vi "State Machine Kernel.vi"(4 "Init?":bool, 5 "Inputs":T4 {"Kobuki Sensors"."Charger Source" items=["DISCHARGING"=0, "DOCKING_CHARGED"=2, "DOCKING_CHARGING"=6, "ADAPTER_CHARGED"=18, "ADAPTER_CHARGING"=22]; "accelerometer"."z axis (g)" format="%.3f"; "accelerometer"."y axis (g)" format="%.3f"; "accelerometer"."x axis (g)" format="%.3f"}, 7 "StateData In":T1) -> (0 "Terminated?":bool, 2 "Outputs":T3, 3 "StateData Out":T1)   [LabVIEW 2017]
uses:
  controls/Inputs.ctl
  shared/Accelerometer.ctl
  Kobuki/KobukiSensors.ctl
  Kobuki/Kobuki Bumps and WheelDrops.ctl
  Kobuki/Kobuki Buttons.ctl
  controls/Outputs.ctl
  controls/StateData.ctl
  controls/StatesEnum.ctl
panel:
  # "Electrical: charging, battery, OI mode"
  # "Sensors: bump, cliff, button, wheel drop"
  # "Motors:"
  # "Inertia"
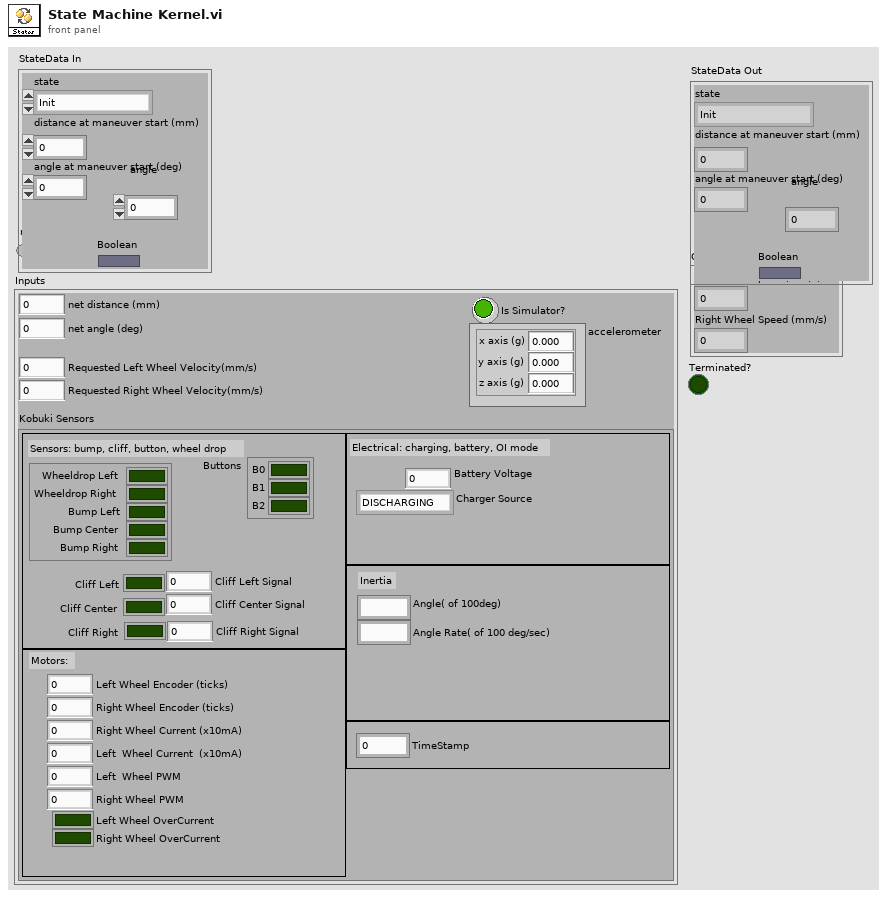
[diagram p1: front panel]
types:
  T1 = typedef "StateData.ctl" = cluster{"distance at maneuver start (mm)":i32, "angle at maneuver start (deg)":i32, "state":T2, "Boolean":bool, "angle":i32}
  T2 = typedef "StatesEnum.ctl" = enum16{"Init", "Center Cliff\n", "Pause", "Drive", "U.Turn", "L.Cliff", "R.Cliff", "Shut", "L.Bump", "R.Bump"}
  T3 = typedef "Outputs.ctl" = cluster{"Left Wheel Speed (mm/s)":i16, "Right Wheel Speed (mm/s)":i16}
  T4 = typedef "Inputs.ctl" = cluster{"net distance (mm)":i32, "net angle (deg)":i32, "accelerometer":T5, "Is Simulator?":bool, "Kobuki Sensors":T6, "Requested Left Wheel Velocity(mm/s)":i32, "Requested Right Wheel Velocity(mm/s)":i32}
  T5 = typedef "Accelerometer.ctl" = cluster{"x axis (g)":dbl, "y axis (g)":dbl, "z axis (g)":dbl}
  T6 = typedef "KobukiSensors.ctl" = cluster{"Bumps + Wheel Drops":T7, "Cliff Left":bool, "Cliff Center":bool, "Cliff Right":bool, "Cliff Left Signal":u16, "Cliff Center Signal":u16, "Cliff Right Signal":u16, "Buttons":T8, "Left Wheel Encoder (ticks)":u16, "Right Wheel Encoder (ticks) ":u16, "Left  Wheel PWM":i8, "Right Wheel PWM":i8, "Left Wheel OverCurrent":bool, "Right Wheel OverCurrent ":bool, "Right Wheel Current (x10mA)":i16, "Left  Wheel Current  (x10mA)":i16, "TimeStamp":u16, "Battery Voltage":dbl, "Angle( of 100deg)":i16, "Angle Rate( of 100 deg/sec)":i16, "Charger Source ":i8}
  T7 = typedef "Kobuki Bumps and WheelDrops.ctl" = cluster{"Wheeldrop Left":bool, "Wheeldrop Right":bool, "Bump Left":bool, "Bump Center":bool, "Bump Right":bool}
  T8 = typedef "Kobuki Buttons.ctl" = cluster{"B0":bool, "B1":bool, "B2":bool}
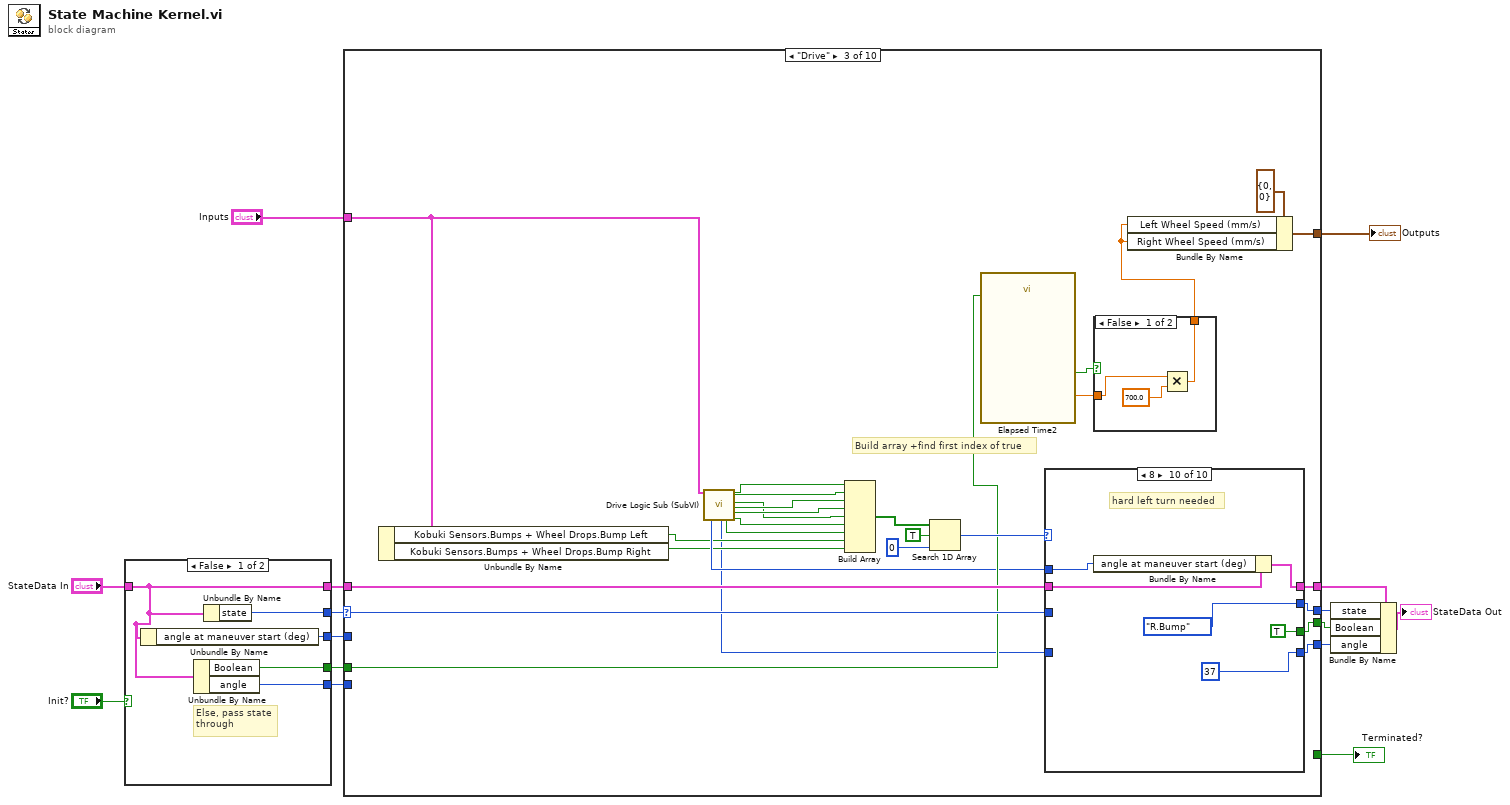
[diagram p0: block diagram]
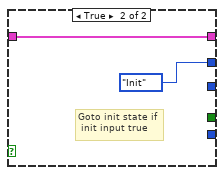
[diagram p2: hidden frame]
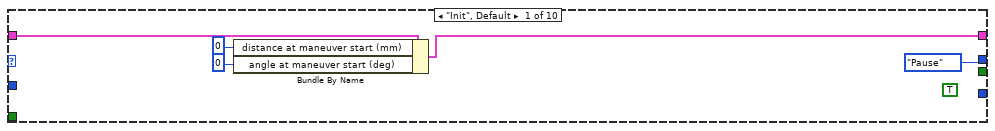
[diagram p3: hidden frame]
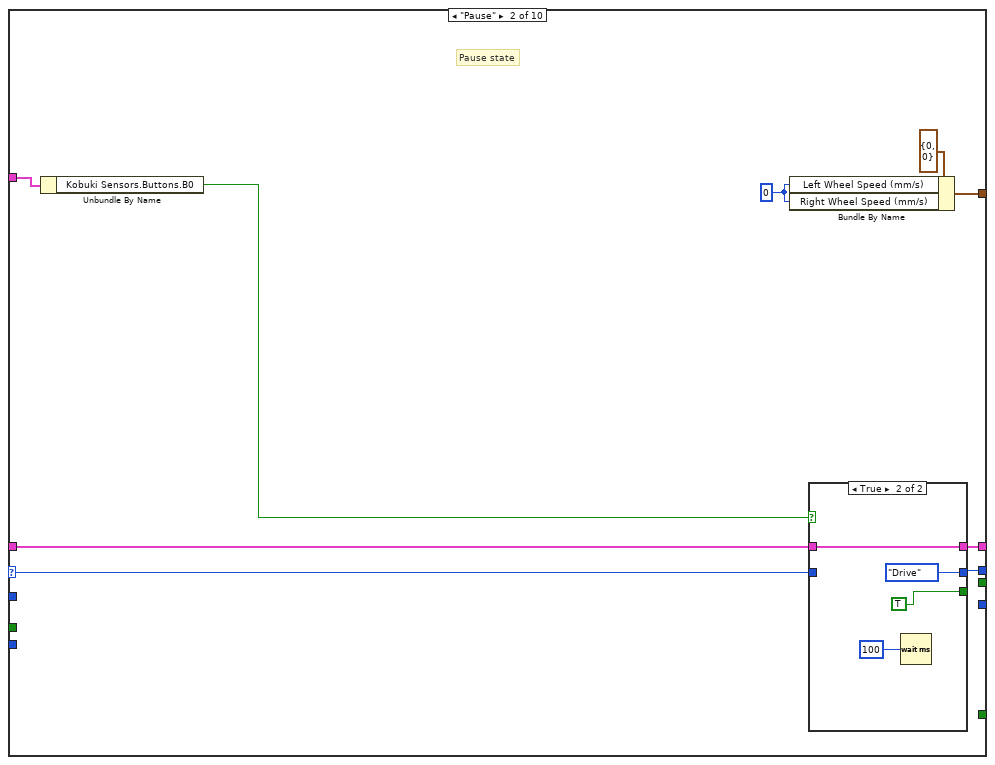
[diagram p4: hidden frame]
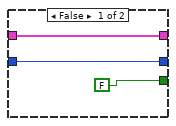
[diagram p5: hidden frame]
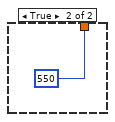
[diagram p6: hidden frame]
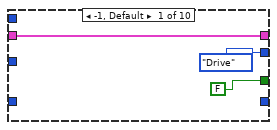
[diagram p7: hidden frame]
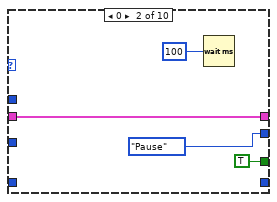
[diagram p8: hidden frame]
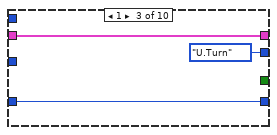
[diagram p9: hidden frame]
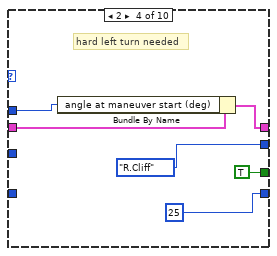
[diagram p10: hidden frame]
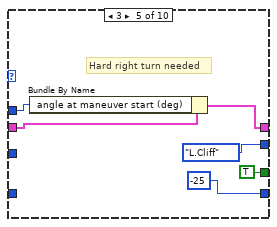
[diagram p11: hidden frame]
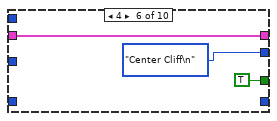
[diagram p12: hidden frame]
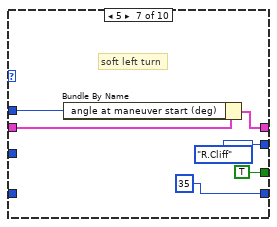
[diagram p13: hidden frame]
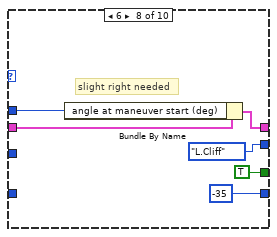
[diagram p14: hidden frame]
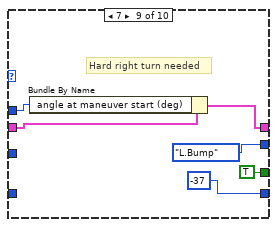
[diagram p15: hidden frame]
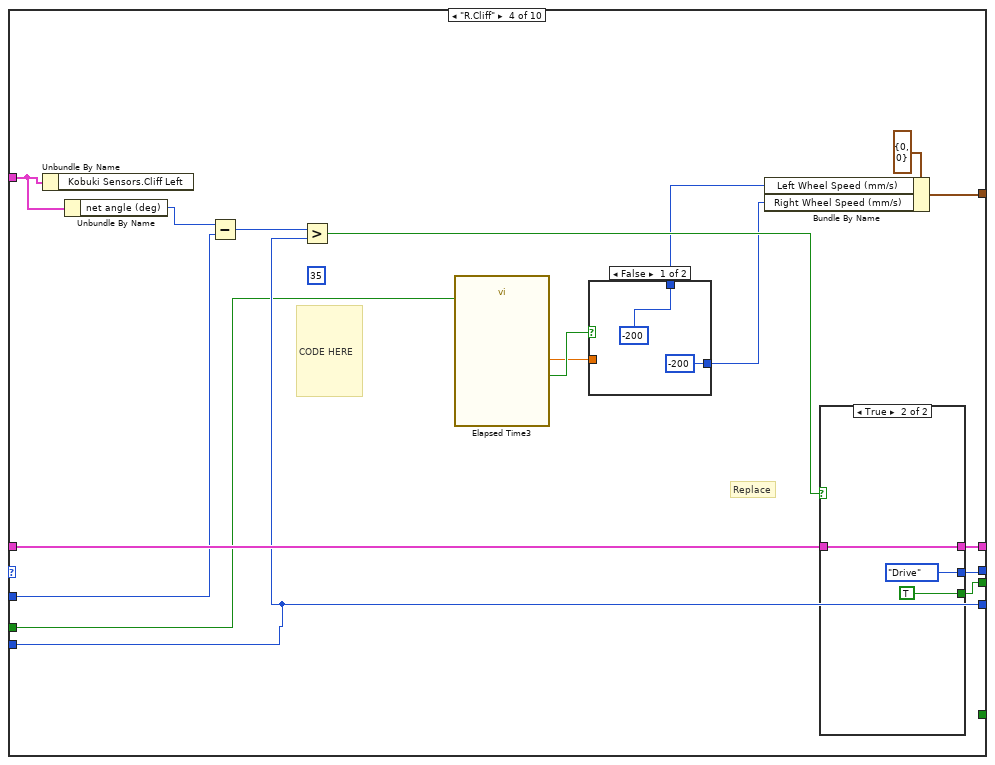
[diagram p16: hidden frame]
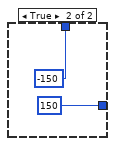
[diagram p17: hidden frame]
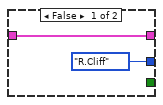
[diagram p18: hidden frame]
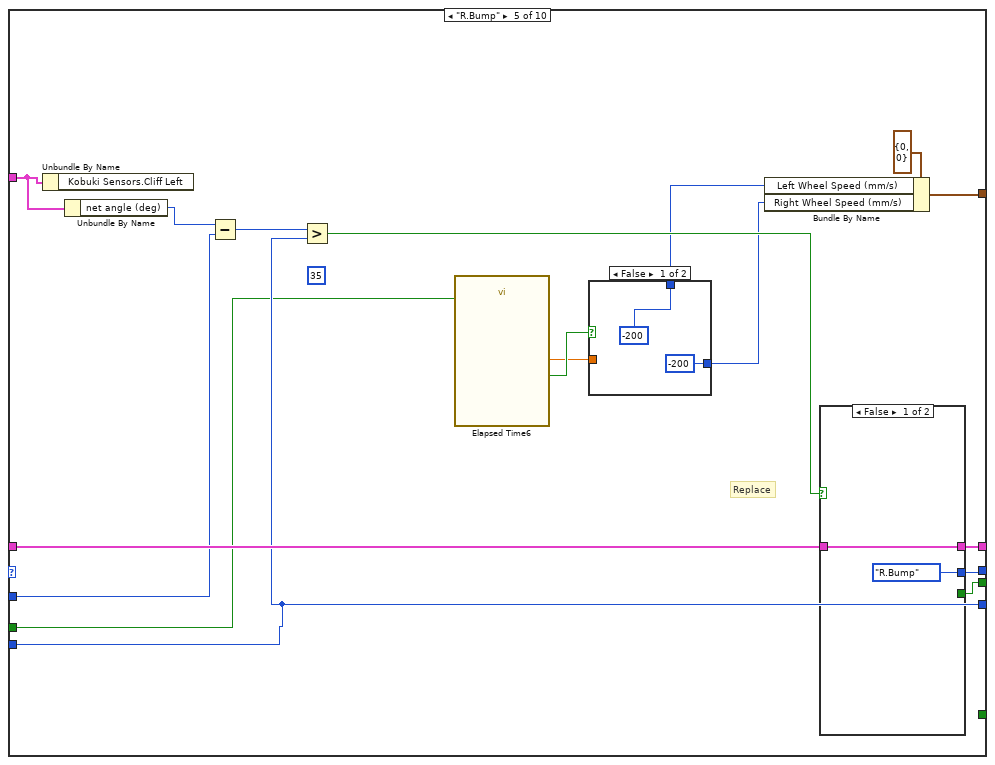
[diagram p19: hidden frame]
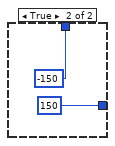
[diagram p20: hidden frame]
diagram:
  n1 = case shown="False" "Init?" {
    tunnel: [w20 StatesEnum."Init" ("StateIn")] -> w13
    tunnel: "StateData In" -> [w18 w21]
    tunnel: [w18 w21] -> w9
    tunnel: [w19 _] -> w6
    tunnel: [w17 _] -> w5
    tunnel: [w16 _] -> w2
    frame False {
      # "Else, pass state \nthrough"
      n2 = Unbundle By Name(w18) -> ("angle at maneuver start (deg)"=w19:i32)
      n3 = Unbundle By Name(w18) -> ("Boolean"=w17:bool, "angle"=w16:i32)
      n4 = Unbundle By Name(w18) -> ("state"=w20:T2)
    }
    frame True {
      # "Goto init state if\n init input true"
    }
  }
  n5 = case shown="\"Drive\"" w13 {
    selector: w13 -> [_ w32 w71 _ _ _ _ _ _ w287]
    tunnel: "Inputs" -> [_ w33 w47 w135 w161 w189 w218 w246 w272 _]
    tunnel: [_ w36 w69 w140 w166 w192 w221 w244 w275 w290] -> w11
    tunnel: [_ _ _ _ _ _ _ _ _ TRUE] -> w12
    tunnel: w9 -> [w27 w30 w64 w138 w164 w190 w219 w242 w273 w288]
    tunnel: [w26 w29 w63 w139 w165 w191 w220 w241 w274 w288] -> w8
    tunnel: w6 -> [_ _ _ w134 w160 w187 w216 _ w270 _]
    tunnel: w5 -> [_ _ w62 w127 w153 w179 w208 w235 _ _]
    tunnel: [_ _ w57 w131 w157 w183 w212 w240 w267 _] -> w4
    tunnel: [StatesEnum."Pause" ("StateIn") w28 w58 w132 w158 w184 w213 w239 w268 w287] -> w3
    tunnel: w2 -> [_ _ _ w130 w156 w182 w211 _ w260 _]
    tunnel: [_ _ w56 w130 w156 w182 w211 _ w260 _] -> w1
    frame "Init", Default {
      (unwired) TRUE
      n6 = Bundle By Name(cluster=w27, "distance at maneuver start (mm)"=0, "angle at maneuver start (deg)"=0) -> (w26:T1)
    }
    frame "Pause" {
      w35 = i16 0 ("Left Wheel Speed (mm/s)")
      # "Pause state"
      n7 = Unbundle By Name(w33) -> ("Kobuki Sensors.Buttons.B0"=w34:bool)
      n8 = Bundle By Name(cluster=T3 {"Left Wheel Speed (mm/s)"=0, "Right Wheel Speed (mm/s)"=0} ("Outputs"), "Left Wheel Speed (mm/s)"=w35, "Right Wheel Speed (mm/s)"=w35) -> (w36:T3)
      n9 = case shown="True" w34 {
        tunnel: w32 -> [w39 _]
        tunnel: [w39 StatesEnum."Drive" ("StateIn")] -> w28
        tunnel: w30 -> [w38 w41]
        tunnel: [w38 w41] -> w29
        tunnel: [FALSE TRUE] -> _
        frame False {
        }
        frame True {
          n10 = Wait (ms)(milliseconds to wait=u32 100) -> ()  [unwired: 1 out]
        }
      }
    }
    frame "Drive" {
      # "Build array +find first index of true"
      n11 = Unbundle By Name(w47) -> ("Kobuki Sensors.Bumps + Wheel Drops.Bump Left"=w46:bool, "Kobuki Sensors.Bumps + Wheel Drops.Bump Right"=w45:bool)
      n12 = call "Drive Logic Sub (SubVI).vi"("Inputs"=w47) -> ("net angle (deg)"=w55:i32, "U-turn Angle"=w44:i32, "Soft Left Cliff"=w48:bool, "Pause"=w54:bool, "U.Turn"=w53:bool, "Center"=w50:bool, "Hard Right Cliff"=w52:bool, "Hard Left Cliff"=w51:bool, "Soft Right Cliff"=w49:bool)  [unwired: 10 in]
      n13 = Build Array(w54, w53, w52, w51, w50, w49, w48, w46, w45) -> (w68:bool[])
      n14 = Search 1D Array(1D array=w68, element=TRUE, start index (0)=0) -> (index of element=w65:i32)
      n15 = call "Elapsed Time2"("Reset"=w62) -> ("Elapsed Time (s)"=w60:dbl, "Time has Elapsed"=w61:bool)  [unwired: 11 in, 6 out]
      n16 = case shown="8" w65 {
        tunnel: w71 -> [_ _ _ _ _ _ _ _ _ _]
        tunnel: w64 -> [w78 w81 w85 w87 w94 w99 w106 w112 w115 w120]
        tunnel: [w78 w81 w85 w86 w93 w99 w105 w110 w114 w119] -> w63
        tunnel: w55 -> [_ _ _ w88 w92 _ w104 w111 w113 w121]
        tunnel: [FALSE TRUE _ TRUE TRUE TRUE TRUE TRUE TRUE TRUE] -> w57
        tunnel: [StatesEnum."Drive" ("StateIn") StatesEnum."Pause" ("StateIn") StatesEnum."U.Turn" ("StateIn") StatesEnum."R.Cliff" ("StateIn") StatesEnum."L.Cliff" ("StateIn") StatesEnum."Center Cliff\n" ("StateIn") StatesEnum."R.Cliff" ("StateIn") StatesEnum."L.Cliff" ("StateIn") StatesEnum."L.Bump" ("StateIn") StatesEnum."R.Bump" ("StateIn")] -> w58
        tunnel: [_ _ w83 25 ("angle") -25 ("angle") _ 35 ("angle") -35 ("angle") -37 ("angle") 37 ("angle")] -> w56
        tunnel: w44 -> [_ _ w83 _ _ _ _ _ _ _]
        frame -1, Default {
        }
        frame 0 {
          n17 = Wait (ms)(milliseconds to wait=u32 100) -> ()  [unwired: 1 out]
        }
        frame 1 {
        }
        frame 2 {
          # "hard left turn needed"
          n18 = Bundle By Name(cluster=w87, "angle at maneuver start (deg)"=w88) -> (w86:T1)
        }
        frame 3 {
          # "Hard right turn needed"
          n19 = Bundle By Name(cluster=w94, "angle at maneuver start (deg)"=w92) -> (w93:T1)
        }
        frame 4 {
        }
        frame 5 {
          # "soft left turn"
          n20 = Bundle By Name(cluster=w106, "angle at maneuver start (deg)"=w104) -> (w105:T1)
        }
        frame 6 {
          # "slight right needed"
          n21 = Bundle By Name(cluster=w112, "angle at maneuver start (deg)"=w111) -> (w110:T1)
        }
        frame 7 {
          # "Hard right turn needed"
          n22 = Bundle By Name(cluster=w115, "angle at maneuver start (deg)"=w113) -> (w114:T1)
        }
        frame 8 {
          # "hard left turn needed"
          n23 = Bundle By Name(cluster=w120, "angle at maneuver start (deg)"=w121) -> (w119:T1)
        }
      }
      n24 = case shown="False" w61 {
        tunnel: w60 -> [w73 _]
        tunnel: [w72 550] -> w59
        frame False {
          n25 = Multiply(x=w73, y=700.0) -> (x*y=w72:dbl)
        }
        frame True {
        }
      }
      n26 = Bundle By Name(cluster=T3 {"Left Wheel Speed (mm/s)"=0, "Right Wheel Speed (mm/s)"=0} ("Outputs"), "Left Wheel Speed (mm/s)"=w59, "Right Wheel Speed (mm/s)"=w59) -> (w69:T3)
    }
    frame "R.Cliff" {
      (unwired) 35 ("y")
      # "Replace"
      # "CODE HERE"
      n27 = Unbundle By Name(w135) -> ()  [unwired: 1 out]
      n28 = Unbundle By Name(w135) -> ("net angle (deg)"=w136:i32)
      n29 = Subtract(x=w136, y=w134) -> (x-y=w137:i32)
      n30 = Greater?(x=w137, y=w130) -> (0:w133:bool)
      n31 = call "Elapsed Time3"("Reset"=w127) -> ("Elapsed Time (s)"=w128:dbl, "Time has Elapsed"=w129:bool)  [unwired: 11 in, 6 out]
      n32 = case shown="False" w129 {
        tunnel: w128 -> [_ _]
        tunnel: [-200 150] -> w125
        tunnel: [-200 -150] -> w126
        frame False {
        }
        frame True {
        }
      }
      n33 = Bundle By Name(cluster=T3 {"Left Wheel Speed (mm/s)"=0, "Right Wheel Speed (mm/s)"=0} ("Outputs"), "Left Wheel Speed (mm/s)"=w126, "Right Wheel Speed (mm/s)"=w125) -> (w140:T3)
      n34 = case shown="True" w133 {
        tunnel: [StatesEnum."R.Cliff" ("StateIn") StatesEnum."Drive" ("StateIn")] -> w132
        tunnel: w138 -> [w146 w149]
        tunnel: [w146 w149] -> w139
        tunnel: [_ TRUE ("Boolean")] -> w131
        frame False {
        }
        frame True {
        }
      }
    }
    frame "R.Bump" {
      (unwired) 35 ("y")
      # "Replace"
      n35 = Unbundle By Name(w161) -> ()  [unwired: 1 out]
      n36 = Unbundle By Name(w161) -> ("net angle (deg)"=w162:i32)
      n37 = Subtract(x=w162, y=w160) -> (x-y=w163:i32)
      n38 = Greater?(x=w163, y=w156) -> (0:w159:bool)
      n39 = call "Elapsed Time6"("Reset"=w153) -> ("Elapsed Time (s)"=w154:dbl, "Time has Elapsed"=w155:bool)  [unwired: 11 in, 6 out]
      n40 = case shown="False" w155 {
        tunnel: w154 -> [_ _]
        tunnel: [-200 150] -> w151
        tunnel: [-200 -150] -> w152
        frame False {
        }
        frame True {
        }
      }
      n41 = Bundle By Name(cluster=T3 {"Left Wheel Speed (mm/s)"=0, "Right Wheel Speed (mm/s)"=0} ("Outputs"), "Left Wheel Speed (mm/s)"=w152, "Right Wheel Speed (mm/s)"=w151) -> (w166:T3)
      n42 = case shown="False" w159 {
        tunnel: [StatesEnum."R.Bump" ("StateIn") StatesEnum."Drive" ("StateIn")] -> w158
        tunnel: w164 -> [w172 w175]
        tunnel: [w172 w175] -> w165
        tunnel: [_ TRUE ("Boolean")] -> w157
        frame False {
        }
        frame True {
        }
      }
    }
    frame "L.Cliff" {
      (unwired) -35 ("y")
      n43 = Unbundle By Name(w189) -> ()  [unwired: 1 out]
      n44 = Unbundle By Name(w189) -> ("net angle (deg)"=w188:i32)
      n45 = Subtract(x=w188, y=w187) -> (x-y=w186:i32)
      n46 = Less?(x=w186, y=w182) -> (x < y?=w185:bool)
      n47 = call "Elapsed Time"("Reset"=w179) -> ("Elapsed Time (s)"=w180:dbl, "Time has Elapsed"=w181:bool)  [unwired: 11 in, 6 out]
      n48 = case shown="True" w181 {
        tunnel: w180 -> [w196 _]
        tunnel: [w194 i16 -150] -> w178
        tunnel: [w194 i16 150] -> w177
        frame False {
          w194 = i16 -200 ("16bit integer")
          n49 = Multiply(x=w196, y=-700.0) -> (x*y=w195:dbl)
          n50 = To Word Integer(number=w195) -> ()  [unwired: 1 out]
        }
        frame True {
        }
      }
      n51 = Bundle By Name(cluster=T3 {"Left Wheel Speed (mm/s)"=0, "Right Wheel Speed (mm/s)"=0} ("Outputs"), "Left Wheel Speed (mm/s)"=w177, "Right Wheel Speed (mm/s)"=w178) -> (w192:T3)
      n52 = case shown="False" w185 {
        tunnel: [StatesEnum."L.Cliff" ("StateIn") StatesEnum."Drive" ("StateIn")] -> w184
        tunnel: w190 -> [w201 w204]
        tunnel: [w201 w204] -> w191
        tunnel: [FALSE ("Boolean") TRUE ("Boolean")] -> w183
        frame False {
        }
        frame True {
        }
      }
    }
    frame "L.Bump" {
      (unwired) -35 ("y")
      n53 = Unbundle By Name(w218) -> ()  [unwired: 1 out]
      n54 = Unbundle By Name(w218) -> ("net angle (deg)"=w217:i32)
      n55 = Subtract(x=w217, y=w216) -> (x-y=w215:i32)
      n56 = Less?(x=w215, y=w211) -> (x < y?=w214:bool)
      n57 = call "Elapsed Time5"("Reset"=w208) -> ("Elapsed Time (s)"=w209:dbl, "Time has Elapsed"=w210:bool)  [unwired: 11 in, 6 out]
      n58 = case shown="True" w210 {
        tunnel: w209 -> [w225 _]
        tunnel: [w223 i16 -150] -> w207
        tunnel: [w223 i16 150] -> w206
        frame False {
          w223 = i16 -200 ("16bit integer")
          n59 = Multiply(x=w225, y=-700.0) -> (x*y=w224:dbl)
          n60 = To Word Integer(number=w224) -> ()  [unwired: 1 out]
        }
        frame True {
        }
      }
      n61 = Bundle By Name(cluster=T3 {"Left Wheel Speed (mm/s)"=0, "Right Wheel Speed (mm/s)"=0} ("Outputs"), "Left Wheel Speed (mm/s)"=w206, "Right Wheel Speed (mm/s)"=w207) -> (w221:T3)
      n62 = case shown="False" w214 {
        tunnel: [StatesEnum."L.Bump" ("StateIn") StatesEnum."Drive" ("StateIn")] -> w213
        tunnel: w219 -> [w230 w233]
        tunnel: [w230 w233] -> w220
        tunnel: [FALSE ("Boolean") TRUE ("Boolean")] -> w212
        frame False {
        }
        frame True {
        }
      }
    }
    frame "Center Cliff\n" {
      w243 = i16 -150 ("Left Wheel Speed (mm/s)")
      n63 = Unbundle By Name(w246) -> ()  [unwired: 5 out]
      n64 = call "Elapsed Time4"("Reset"=w235) -> ("Elapsed Time (s)"=w237:dbl, "Time has Elapsed"=w238:bool)  [unwired: 11 in, 6 out]
      n65 = case shown="True" w238 {
        tunnel: w237 -> [_ _]
        tunnel: [-200 150] -> _
        tunnel: [-200 -150] -> _
        tunnel: [FALSE TRUE] -> w236
        frame False {
        }
        frame True {
        }
      }
      n66 = case shown="False" w236 {
        tunnel: w242 -> [w254 w258]
        tunnel: [w254 w258] -> w241
        tunnel: [FALSE ("Boolean") TRUE ("Boolean")] -> w240
        tunnel: [StatesEnum."Center Cliff\n" ("StateIn") StatesEnum."Drive" ("StateIn")] -> w239
        frame False {
        }
        frame True {
        }
      }
      n67 = Bundle By Name(cluster=T3 {"Left Wheel Speed (mm/s)"=0, "Right Wheel Speed (mm/s)"=0} ("Outputs"), "Left Wheel Speed (mm/s)"=w243, "Right Wheel Speed (mm/s)"=w243) -> (w244:T3)
    }
    frame "U.Turn" {
      n68 = Unbundle By Name(w272) -> ("net angle (deg)"=w271:i32)
      n69 = Subtract(x=w271, y=w270) -> (x-y=w262:i32)
      n70 = Absolute Value(x=w262) -> (abs(x)=w261:i32)
      n71 = Absolute Value(x=w260) -> (abs(x)=w259:i32)
      n72 = Greater?(x=w260, y=0) -> (0:w263:bool)
      n73 = Greater?(x=w261, y=w259) -> (0:w269:bool)
      n74 = case shown="False" w263 {
        tunnel: [i16 -150 i16 150] -> w266
        tunnel: [i16 150 i16 -150] -> w265
        frame False {
        }
        frame True {
        }
      }
      n75 = Bundle By Name(cluster=T3 {"Left Wheel Speed (mm/s)"=0, "Right Wheel Speed (mm/s)"=0} ("Outputs"), "Left Wheel Speed (mm/s)"=w265, "Right Wheel Speed (mm/s)"=w266) -> (w275:T3)
      n76 = case shown="False" w269 {
        tunnel: [StatesEnum."U.Turn" ("StateIn") StatesEnum."Drive" ("StateIn")] -> w268
        tunnel: w273 -> [w282 w285]
        tunnel: [w282 w285] -> w274
        tunnel: [FALSE ("Boolean") TRUE ("Boolean")] -> w267
        frame False {
        }
        frame True {
        }
      }
    }
    frame "Shut" {
      w291 = i16 0 ("Left Wheel Speed (mm/s)")
      # "Shutdown"
      n77 = Bundle By Name(cluster=T3 {"Left Wheel Speed (mm/s)"=0, "Right Wheel Speed (mm/s)"=0} ("Outputs"), "Left Wheel Speed (mm/s)"=w291, "Right Wheel Speed (mm/s)"=w291) -> (w290:T3)
    }
  }
  "Terminated?" <- w12
  "Outputs" <- w11
  n78 = Bundle By Name(cluster=w8, "state"=w3, "Boolean"=w4, "angle"=w1) -> (→"StateData Out":T1)
